vi "GT_InitLookAhead.vi"(5 "accMax":dbl, 7 "T":dbl, 8 "n":i16, 9 "fifo in":i16, 10 "crd in":i16, 11 "rtn_In":cluster{"rtn":i16, "Func":string}) -> (0 "MemorySpace":T2(array[cluster]), 1 "fifo out":i16, 2 "crd out":i16, 3 "rtn_Out":cluster{"rtn":i16, "Func":string})   [LabVIEW 2014]
uses:
  VC6/gts.dll
panel:
  in  "Initl":T1
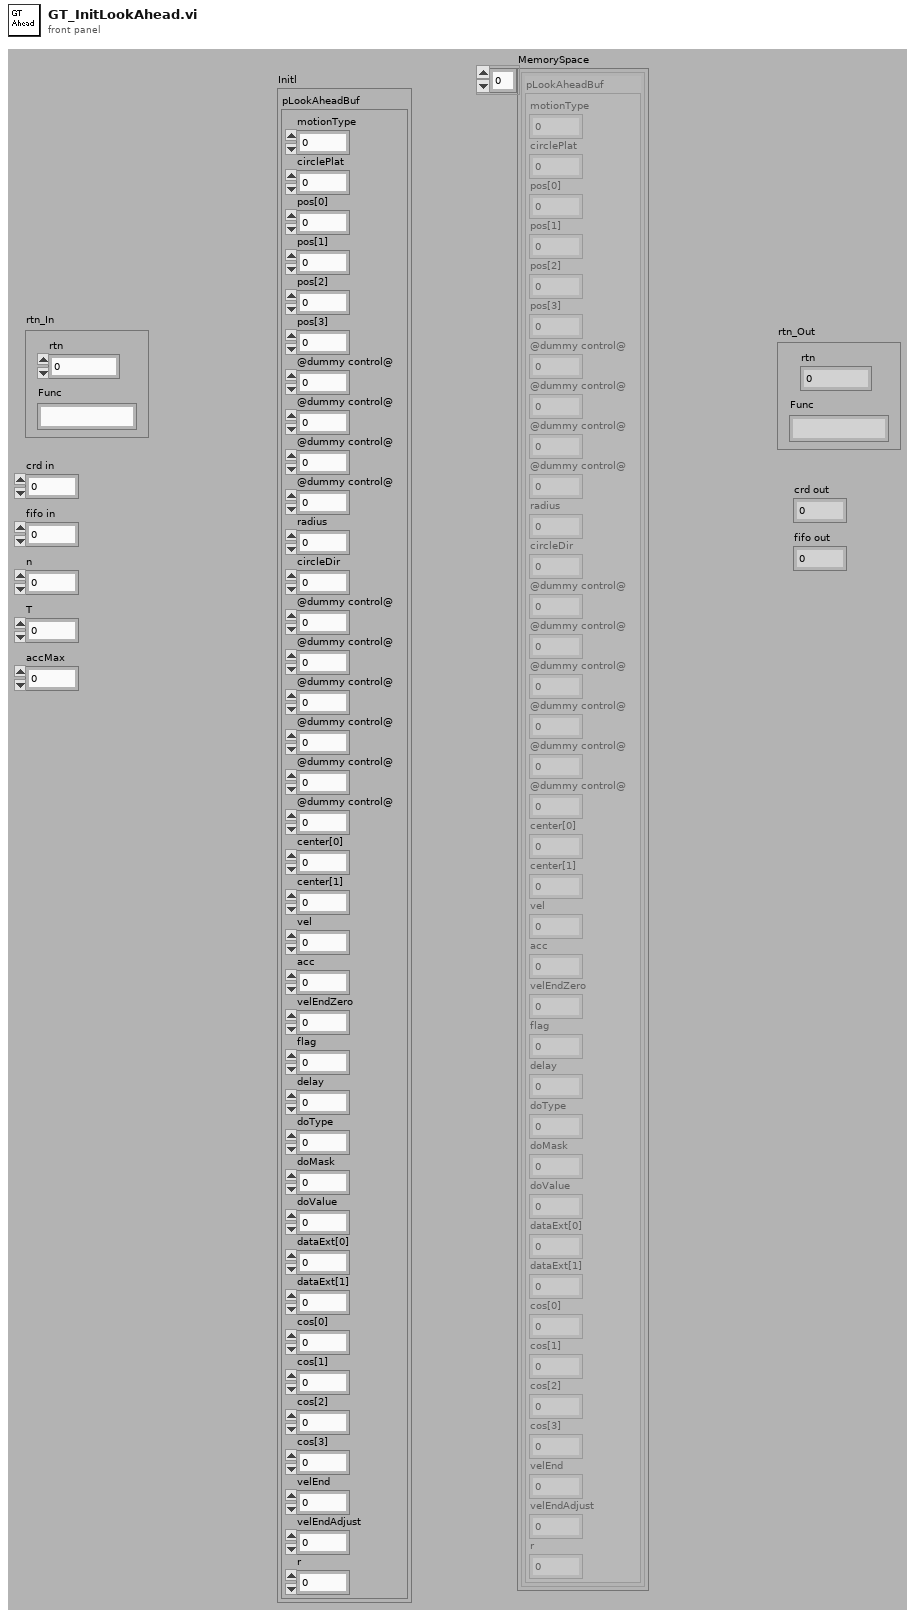
[diagram p1: front panel]
types:
  T1 = cluster{"pLookAheadBuf":cluster{"motionType":i16, "circlePlat":i16, "pos[0]":i32, "pos[1]":i32, "pos[2]":i32, "pos[3]":i32, "@dummy control@":i8, "@dummy control@":i8, "@dummy control@":i8, "@dummy control@":i8, "radius":dbl, "circleDir":i16, "@dummy control@":i8, "@dummy control@":i8, "@dummy control@":i8, "@dummy control@":i8, "@dummy control@":i8, "@dummy control@":i8, "center[0]":dbl, "center[1]":dbl, "vel":dbl, "acc":dbl, "velEndZero":i16, "flag":i16, "delay":u16, "doType":i16, "doMask":u16, "doValue":u16, "dataExt[0]":u16, "dataExt[1]":u16, "cos[0]":dbl, "cos[1]":dbl, "cos[2]":dbl, "cos[3]":dbl, "velEnd":dbl, "velEndAdjust":dbl, "r":dbl}}
  T2 = cluster{"pLookAheadBuf":cluster{"motionType":i16, "circlePlat":i16, "pos[0]":i32, "pos[1]":i32, "pos[2]":i32, "pos[3]":i32, "@dummy control@":i8, "@dummy control@":i8, "@dummy control@":i8, "@dummy control@":i8, "radius":dbl, "circleDir":i16, "@dummy control@":i8, "@dummy control@":i8, "@dummy control@":i8, "@dummy control@":i8, "@dummy control@":i8, "@dummy control@":i8, "center[0]":dbl, "center[1]":dbl, "vel":dbl, "acc":dbl, "velEndZero":i16, "flag":i16, "delay":u16, "doType":i16, "doMask":u16, "doValue":u16, "dataExt[0]":u16, "dataExt[1]":u16, "cos[0]":dbl, "cos[1]":dbl, "cos[2]":dbl, "cos[3]":dbl, "velEnd":dbl, "velEndAdjust":dbl, "r":dbl}}[]
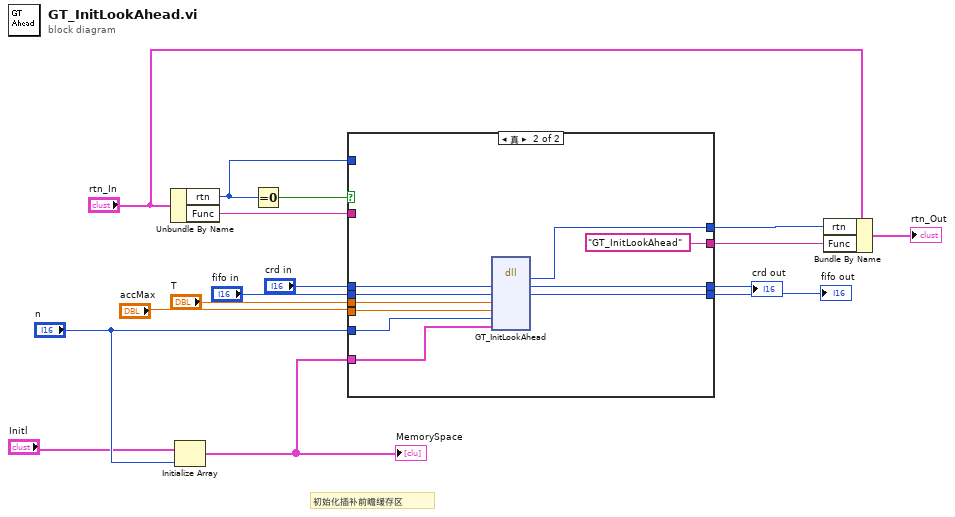
[diagram p0: block diagram]
diagram:
  # "初始化插补前瞻缓存区"
  n1 = Unbundle By Name("rtn_In") -> ("rtn"=w4:i16, "Func"=w3:string)
  n2 = Initialize Array("Initl", "n") -> (w1:T2)
  "MemorySpace" <- w1
  n3 = Equal To 0?(x=w4) -> (x = 0?=w16:bool)
  n4 = case shown="真" w16 {
    tunnel: [w20 w30] -> w13
    tunnel: [w19 "GT_InitLookAhead" ("Func")] -> w12
    tunnel: "crd in" -> [w18 w28]
    tunnel: [w18 w27] -> w10
    tunnel: "fifo in" -> [w17 w26]
    tunnel: [w17 w25] -> w8
    tunnel: "T" -> [_ w24]
    tunnel: "accMax" -> [_ w23]
    tunnel: "n" -> [_ w22]
    tunnel: w1 -> [_ w21]
    tunnel: w4 -> [w20 _]
    tunnel: w3 -> [w19 _]
    frame False {
    }
    frame True {
      n5 = dll-call lib="PTH2Fabs DNewGTS AC-800LWin7版源程序-20170926gts85VC6gts.dll" fn="GT_InitLookAhead"("crd"=w28, "fifo"=w26, "T"=w24, "accMax"=w23, "n"=w22, "pLookAheadBuf"=w21) -> ("rtn"=w30:i16, "crd"=w27:i16, "fifo"=w25:i16)  [unwired: 7 in, 2 out]
    }
  }
  "crd out" <- w10
  "fifo out" <- w8
  n6 = Bundle By Name(cluster="rtn_In", "rtn"=w13, "Func"=w12) -> (→"rtn_Out":cluster{"rtn":i16, "Func":string})
